vi "Read TimeStamp.vi"(8 "error in (no error)":errorcluster, 11 "DataToSend in":refnum<class "DataToSend.lvclass">) -> (0 "error out":errorcluster, 2 "TimeStamp":timestamp, 3 "DataToSend out":refnum<class "DataToSend.lvclass">)   [LabVIEW 2022 SP3, in "TcpServer.lvlib" / "DataToSend.lvclass"]
uses:
  DataToSend.lvclass
  DataToSend.lvclass/DataToSend.ctl
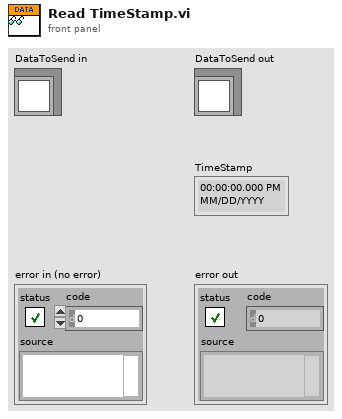
[diagram p1: front panel]
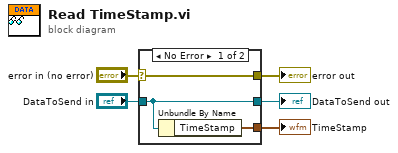
[diagram p0: block diagram]
diagram:
  n1 = case shown="No Error" "error in (no error)" {
    selector: "error in (no error)" -> [w8 w9]
    tunnel: [w8 w9] -> w4
    tunnel: [w7 w10] -> w2
    tunnel: "DataToSend in" -> [w7 w10]
    tunnel: [w6 _] -> w1
    frame No Error {
      n2 = Unbundle By Name(w7) -> ("TimeStamp"=w6:timestamp)
    }
    frame Error {
    }
  }
  "error out" <- w4
  "DataToSend out" <- w2
  "TimeStamp" <- w1
